vi "ProcessTemplate (TimedLoop).vi"   [LabVIEW 2021]
uses:
  SMO/SMO.lvclass
  <vilib>/Platform/TimedLoop/XDataNode/wakeup.ctl
  <vilib>/Platform/TimedLoop/XDataNode/XDNodeRunTimeDep.lvlib
  <vilib>/Platform/TimedLoop/XDataNode/nitl_modes.ctl
  <vilib>/Platform/TimedLoop/XDataNode/timing_clust.ctl
  <vilib>/platform/TimedLoop/XDataNode/XDataNode.xnode
types:
  T1 = typedef "XDNodeRunTimeDep.lvlib/timing_clust.ctl" = cluster{"Expected End [f-1]":u64, "Actual End [f-1]":u64, "Finished Late? [f-1]":bool, "Expected End [i-1]":u64, "Actual End [i-1]":u64, "Finished Late? [i-1]":bool, "Expected Start [i]":u64, "Actual Start [i]":u64, "Expected Start [f]":u64, "Actual Start [f]":u64, "Source Name":string, "Structure Name":string, "Period":i64, "Deadline":i64, "Offset":i64, "Start":i64, "Priority":i32, "Timeout":i32, "Mode":T2, "Wakeup Reason":T3, "Error":errorcluster, "Source Type":string, "Secondary Source Type":string, "Global End Time":u64, "Global Start Time":u64, "Frame Duration":u64, "Iteration Duration":u64, "Assigned CPU":i32, "I/O Scan Engine Mode":u32}
  T2 = typedef "XDNodeRunTimeDep.lvlib/nitl_modes.ctl" = enum32{"No Change", "Process missed periods, maintain original phase", "Discard missed periods, maintain original phase", "Process missed periods, ignore original phase", "Discard missed periods, ignore original phase"}
  T3 = typedef "XDNodeRunTimeDep.lvlib/wakeup.ctl" = enum32{"Normal", "Aborted", "Asynchronous wakeup", "Timing source error", "Timed loop error", "Timeout"}
  T4 = typedef "smo.lvlib/SMO.lvclass/Protected Events.ctl" = cluster{"StopProcesses":refnum<user-event>, "AbortProcesses":refnum<user-event>, "Config Changed":refnum<user-event>, "Dependency":refnum<user-event>}
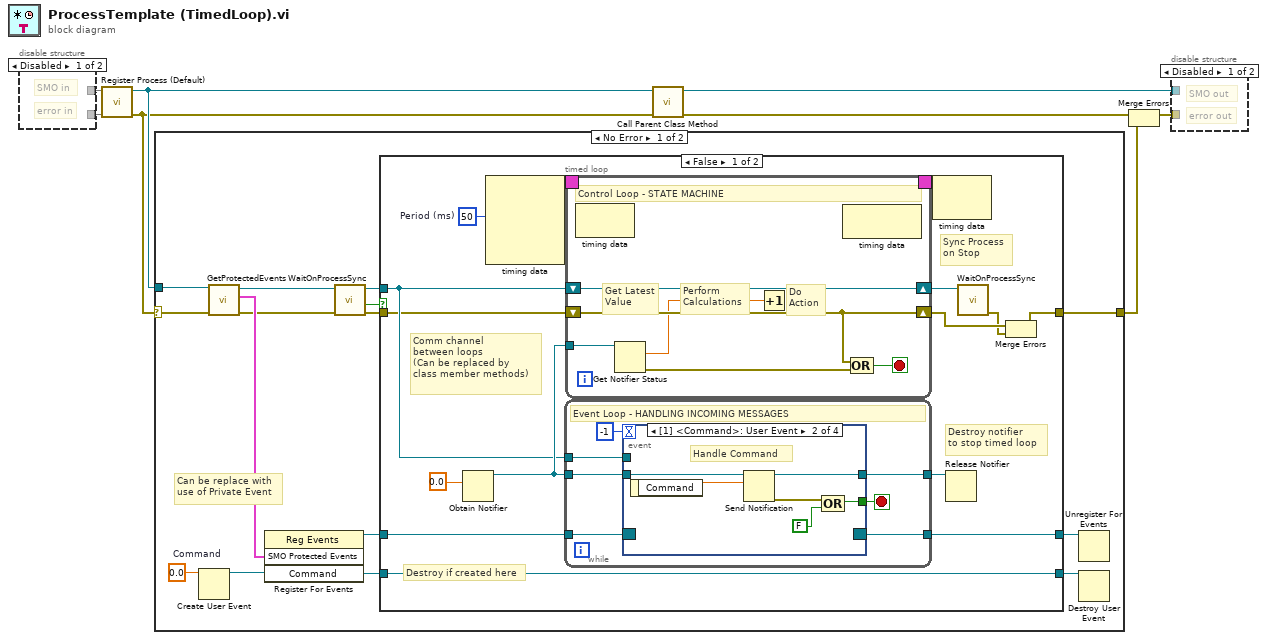
[diagram p0: block diagram]
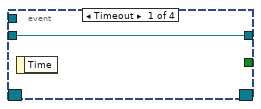
[diagram p4: hidden frame]
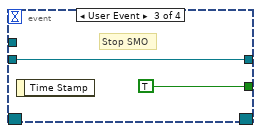
[diagram p5: hidden frame]
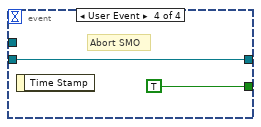
[diagram p6: hidden frame]
diagram:
  n1 = disable-structure shown="Disabled" {
    disable-tunnel: [_ _] -> w2
    disable-tunnel: [_ _] -> w1
    frame Disabled {
      # "error in"
      # "SMO in"
    }
    frame Enabled {
    }
  }
  n2 = call "Register Process (Default).vi"("error in (no error)"=w2, "SMO"=w1) -> ("error out"=w3:errorcluster, "SelfRef"=w4:refnum<class "SMO.lvclass">)  [unwired: 8 in]
  n3 = case shown="No Error" w3 {
    selector: w3 -> [w18 w71]
    tunnel: w4 -> [w21 _]
    tunnel: [w14 w71] -> w7
    frame No Error {
      w11 = 0.0  # Command
      # "Can be replace with\nuse of Private Event"
      n4 = Create User Event(user event datatype=w11) -> (user event=w10:refnum<user-event>)  [unwired: 1 in, 1 out]
      n5 = call "GetProtectedEvents.vi"("error in (no error)"=w18, "SMO"=w21) -> ("error out"=w19:errorcluster, "SMO Protected Events"=w22:T4, "SMO out"=w20:refnum<class "SMO.lvclass">)  [unwired: 7 in]
      n6 = register-events(w22, w10) -> (reference out=w12:refnum<event-registration>)  [unwired: 2 in, 1 out]
      n7 = call "WaitOnProcessSync.vi"("error in (no error)"=w19, "SMO"=w20) -> ("error out"=w16:errorcluster, "Don't run?"=w15:bool, "SMO out"=w17:refnum<class "SMO.lvclass">)  [unwired: 7 in]
      n8 = case shown="False" w15 {
        tunnel: w16 -> [w27 w69]
        tunnel: w17 -> [w28 _]
        tunnel: w12 -> [w33 w70]
        tunnel: [w23 w69] -> w14
        tunnel: [w32 w70] -> w13
        tunnel: [w26 w68] -> w9
        tunnel: w10 -> [w26 w68]
        frame False {
          w35 = i64 50  # Period (ms)
          # "Destroy if created here"
          # "Destroy notifier\nto stop timed loop"
          # "Comm channel\nbetween loops\n(Can be replaced by\nclass member methods)"
          # "Sync Process\non Stop"
          n9 = Obtain Notifier(notification data type=0.0 ("Setpoint")) -> (notifier out=w29:refnum<notifier>)  [unwired: 3 in, 2 out]
          n10 = node-c288(w35) -> (w37:T1)  [unwired: 3 in]
          n11 = while {
            tunnel: w33 -> [w43]
            tunnel: [w42] -> w32
            tunnel: [w39] -> w31
            tunnel: w29 -> [w40]
            tunnel: w28 -> [w38]
            stop <- w41 stop-if-true
            # "Event Loop - HANDLING INCOMING MESSAGES"
            n12 = event shown="[1] <Command>: User Event" {
              selector: w43 -> [_ _ _ _]
              dyn-events: [_ _ _ _] -> w42
              timeout: -1 -> [_ _ _ _]
              tunnel: [_ w47 TRUE TRUE] -> w41
              tunnel: w40 -> [w45 w51 w52 w54]
              tunnel: [w45 w50 w52 w54] -> w39
              tunnel: w38 -> [_ _ _ _]
              event Timeout {
                n13 = event-data() -> ()  [unwired: 1 in, 1 out]
              }
              event User Event {
                # "Handle Command"
                n14 = event-data() -> ("Command"=w49:dbl)  [unwired: 1 in]
                n15 = Send Notification(notification=w49, notifier=w51) -> (notifier out=w50:refnum<notifier>, error out=w48:errorcluster)  [unwired: 1 in]
                n16 = Compound Arithmetic op=OR(w48, FALSE) -> (w47:bool)
              }
              event User Event {
                # "Stop SMO"
                n17 = event-data() -> ()  [unwired: 1 in, 1 out]
              }
              event User Event {
                # "Abort SMO"
                n18 = event-data() -> ()  [unwired: 1 in, 1 out]
              }
            }
          }
          n19 = timed-loop {
            timing: w37 -> [_]
            timing-out: [_] -> w36
            tunnel: w29 -> [w61]
            shift-right: [w58] -> w34
            shift-left: w28 -> [w58]
            shift-right: [w57] -> w25
            shift-left: w27 -> [w57]
            stop <- w59 stop-if-true
            # "Do\nAction"
            # "Perform \nCalculations"
            # "Get Latest\nValue"
            # "Control Loop - STATE MACHINE"
            n20 = node-c288() -> ()  [unwired: 1 in, 1 out]
            n21 = Get Notifier Status(notifier=w61) -> (current notification=w56:dbl, error out=w60:errorcluster)  [unwired: 1 in, 3 out]
            n22 = Increment(x=w56) -> ()  [unwired: 1 out]
            n23 = node-c288() -> ()  [unwired: 1 in, 1 out]
            n24 = Compound Arithmetic op=OR(w57, w60) -> (w59:bool)
          }
          n25 = node-c288(w36) -> ()  [unwired: 1 out]
          n26 = Release Notifier(notifier=w31) -> ()  [unwired: 2 in, 3 out]
          n27 = call "WaitOnProcessSync.vi"("SMO"=w34) -> ("error out"=w24:errorcluster)  [unwired: 8 in, 2 out]
          n28 = Merge Errors(w25, w24) -> (w23:errorcluster)
        }
        frame True {
        }
      }
      n29 = Unregister For Events(event registration refnum=w13) -> ()  [unwired: 1 in, 1 out]
      n30 = Destroy User Event(user event=w9) -> ()  [unwired: 1 in, 1 out]
    }
    frame Error {
    }
  }
  n31 = call-parent "Call Parent Class Method"("error in"=w3, "SMO"=w4) -> ("error out"=w8:errorcluster, "SMO out"=w6:refnum<class "SMO.UI.lvclass">)  [unwired: 8 in]
  n32 = Merge Errors(w8, w7) -> (w5:errorcluster)
  n33 = disable-structure shown="Disabled" {
    disable-tunnel: w6 -> [_ _]
    disable-tunnel: w5 -> [_ _]
    frame Disabled {
      # "error out"
      # "SMO out"
    }
    frame Enabled {
    }
  }
